vi "ArrayFirst_S.vi"(11 "1D Array In":string[](array[string])) -> (2 "Rest of Array":string[](array[string]), 3 "First Element":string)   [LabVIEW 2013]
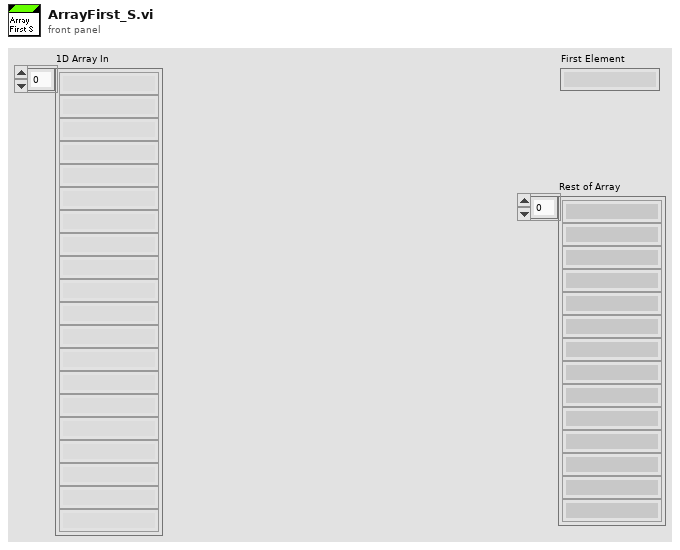
[diagram p1: front panel]
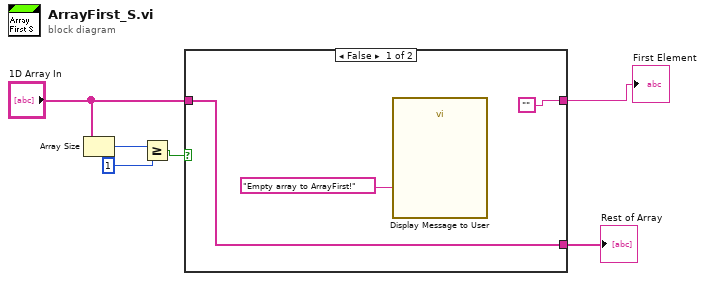
[diagram p0: block diagram]
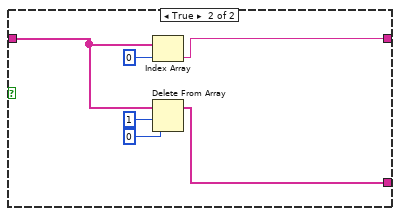
[diagram p2: hidden frame]
diagram:
  n1 = Array Size(array="1D Array In") -> (size(s)=w6:i32)
  n2 = Greater Or Equal?(x=w6, y=1) -> (x >= y?=w4:bool)
  n3 = case shown="False" w4 {
    tunnel: "1D Array In" -> [w9 w11]
    tunnel: ["" w14] -> w1
    tunnel: [w9 w10] -> w2
    frame False {
      n4 = call "Display Message to User"("Message"="Empty array to ArrayFirst!") -> ()  [unwired: 9 in, 2 out]
    }
    frame True {
      n5 = Index Array(array=w11, index=0) -> (element=w14:string)
      n6 = Delete From Array(array=w11, length=1, index=0) -> (array with subset deleted=w10:string[])  [unwired: 1 out]
    }
  }
  "Rest of Array" <- w2
  "First Element" <- w1
